vi "Write Single Numeric To XL.vi"(8 "error in":errorcluster, 9 "Write/Read Cell Numeric":T1 {"Data 1D" format="%.2f"; "Data 2D" format="%.2f"; "1 Data" format="%.2f"}, 11 "Work Sheet 2":refnum<k7>) -> (0 "error out":errorcluster, 3 "Work Sheet":refnum<k7>)   [LabVIEW 2017]
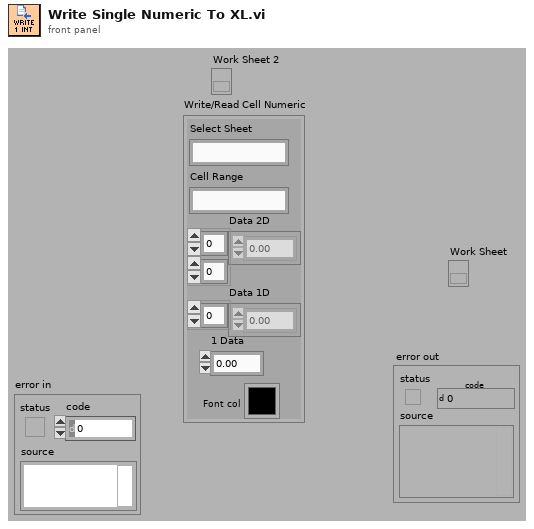
[diagram p1: front panel]
types:
  T1 = cluster{"Cell Range":string, "Select Sheet":string, "1 Data":dbl, "Data 2D":dbl[][], "Data 1D":dbl[], "Font col":u32}
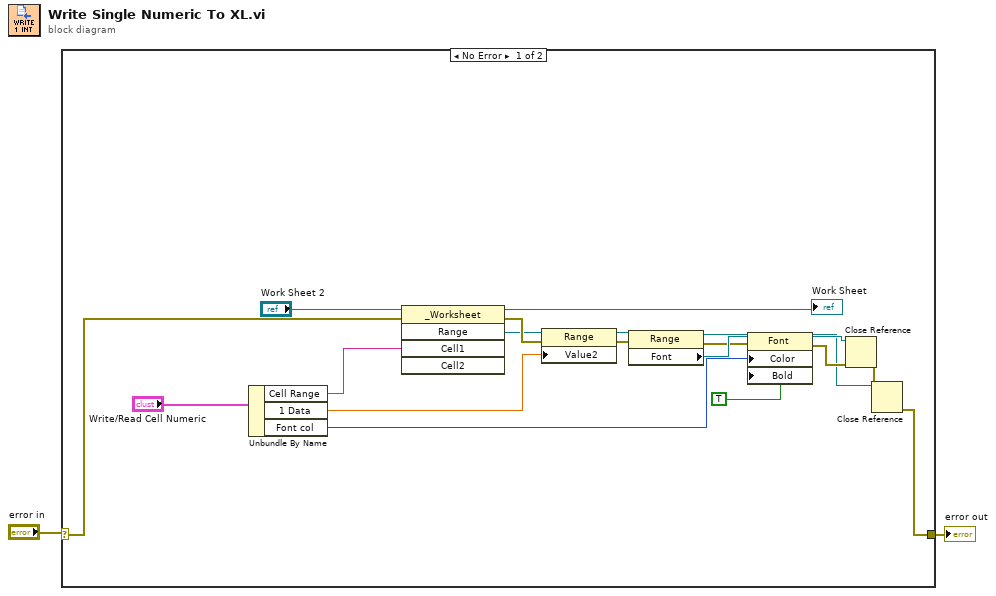
[diagram p0: block diagram]
diagram:
  n1 = case shown="No Error" "error in" {
    selector: "error in" -> [w21 w22]
    tunnel: [w4 w22] -> w1
    frame No Error {
      n2 = Unbundle By Name("Write/Read Cell Numeric") -> ("Cell Range"=w17:string, "1 Data"=w15:dbl, "Font col"=w11:u32)
      n3 = invoke class="_Worksheet" method="Range"(reference="Work Sheet 2", error in=w21, "Cell1"=w17) -> (reference out=→"Work Sheet":refnum<k7>, error out=w20:errorcluster, "Range"=w16:refnum<k7>)  [unwired: 2 in, 2 out]
      n4 = property class="Range"(reference=w16, error in=w20, "Value2"=w15) -> (reference out=w13:refnum<k7>, error out=w9:errorcluster)
      n5 = property class="Range"(reference=w13, error in=w9) -> (reference out=w6:refnum<k7>, error out=w10:errorcluster, "Font"=w12:refnum<k7>)
      n6 = property class="Font"(reference=w12, error in=w10, "Color"=w11, "Bold"=TRUE) -> (reference out=w7:refnum<k7>, error out=w8:errorcluster)
      n7 = Close Reference(reference=w7, error in (no error)=w8) -> (error out=w5:errorcluster)
      n8 = Close Reference(reference=w6, error in (no error)=w5) -> (error out=w4:errorcluster)
    }
    frame Error {
    }
  }
  "error out" <- w1
